vi "Error to System Logger (SubVI).vi"(8 "error in (no error)":errorcluster, 10 "Message Tag":string, 11 "Sys Msg Queue":refnum<queue>) -> (0 "error out":errorcluster)   [LabVIEW 2019]
doc: "Record errors to system log"
uses:
  Globals and Definitions/System Message.ctl
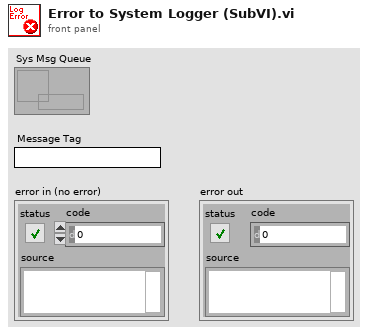
[diagram p1: front panel]
types:
  T1 = typedef "System Message.ctl" = cluster{"Message Tag":string, "Message Body":string, "Snooze Time (s)":dbl, "Snooze Alert?":bool, "Log Event?":bool, "Send Email":i32}
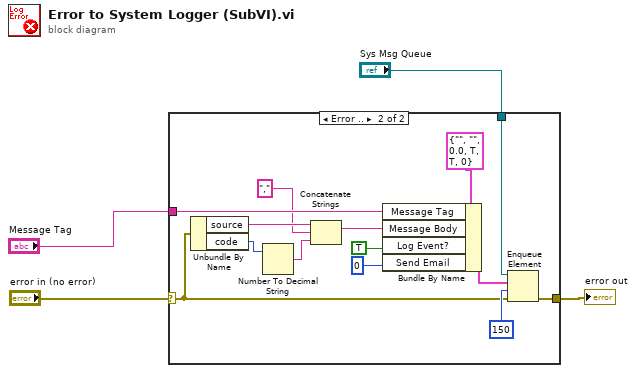
[diagram p0: block diagram]
diagram:
  n1 = case shown="Error .." "error in (no error)" {
    selector: "error in (no error)" -> [w5 w16]
    tunnel: [w5 w15] -> w2
    tunnel: "Sys Msg Queue" -> [_ w13]
    tunnel: "Message Tag" -> [_ w12]
    frame No Error {
    }
    frame Error {
      n2 = Unbundle By Name(w16) -> ("source"=w9:string, "code"=w10:i32)
      n3 = Number To Decimal String(number=w10) -> (decimal integer string=w7:string)  [unwired: 1 in]
      n4 = Concatenate Strings(w9, "," ("string"), w7) -> (w6:string)
      n5 = Bundle By Name(cluster=T1 {"Message Tag"="", "Message Body"="", "Snooze Time (s)"=0.0, "Snooze Alert?"=TRUE, "Log Event?"=TRUE, "Send Email"=0}, "Message Tag"=w12, "Message Body"=w6, "Log Event?"=TRUE, "Send Email"=0) -> (w18:T1)
      n6 = Enqueue Element(queue=w13, element=w18, timeout in ms (-1)=150, error in (no error)=w16) -> (error out=w15:errorcluster)  [unwired: 2 out]
    }
  }
  "error out" <- w2
